vi "insertActions.vi"(7 "before (NULL)":refnum<class "QAction.lvclass">, 8 "Error In":errorcluster, 10 "actions":refnum<class "QAction.lvclass">[](array[class]), 11 "QWidget In":refnum<class "QWidget.lvclass">) -> (0 "Error Out":errorcluster, 3 "QWidget Out":refnum<class "QWidget.lvclass">)   [LabVIEW 2014, in "QWidget.lvclass"]
doc: "LabVIEW-specific documentation is not yet available. See <b>https://doc.qt.io/qt-5/qwidget.html#insertActions</b>"
uses:
  QWidget.lvclass
  QAction/QAction.lvclass
  LQ Core/LQIdentity/LQIdentity.lvclass/LQIdentity.ctl
  LQ Core/LQ Core.lvlib
  LQ Core/LQIdentity/LQIdentity.lvclass
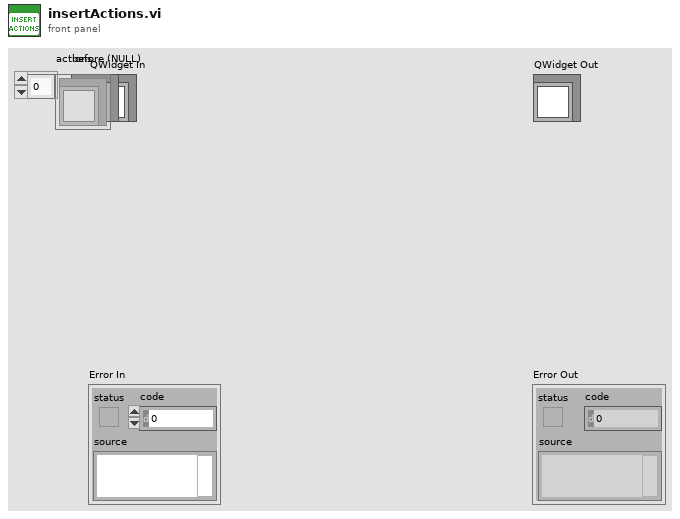
[diagram p1: front panel]
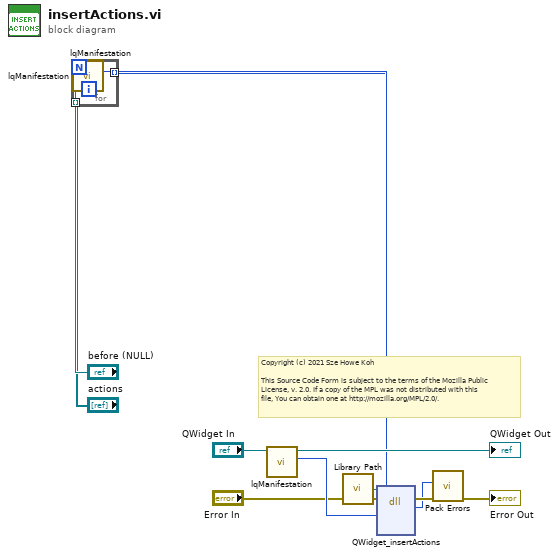
[diagram p0: block diagram]
diagram:
  # "Copyright (c) 2021 Sze Howe Koh\n\nThis Source Code Form is subject to the terms of the Mozilla Public\nLicense, v. 2.0. If a copy of the MPL was not distributed with this\nfile, You can obtain one at http://mozilla.org/MPL/2.0/."
  n1 = for {
    tunnel: "actions" -> [w14] mode=indexing
    tunnel: [w13] -> w1 mode=indexing
    n2 = call "lqManifestation.vi"("LQIdentity in"=w14) -> ("Manifestation"=w13:u64)  [unwired: 9 in, 1 out]
  }
  n3 = call "lqManifestation.vi"("LQIdentity in"="before (NULL)") -> ("Manifestation"=w3:u64)  [unwired: 9 in, 1 out]
  n4 = call "lqManifestation.vi"("LQIdentity in"="QWidget In") -> ("Manifestation"=w9:u64, "LQIdentity out"=→"QWidget Out":refnum<class "QWidget.lvclass">)  [unwired: 9 in]
  n5 = call "Library Path.vi"() -> ("Library Path"=w10:path)
  n6 = dll-call lib="?" fn="QWidget_insertActions"(path in=w10, error in="Error In", "_instance"=w9, "before"=w3, "actions"=w1) -> (error out=w7:errorcluster, w5:i32)  [unwired: 4 in, 1 out]
  n7 = call "Pack Errors.vi"("Error In"=w7, "Error Code"=w5) -> ("Error Out"=→"Error Out":errorcluster)  [unwired: 9 in]
